vi "Main.vi"   [LabVIEW 2017]
doc: "The start-up VI for our application and the UI"
types:
  T1 = typedef "View Model.ctl" = cluster{"Error Model":T2, "Elevator Model":T3, "Configuration Model":T4, "Shared Model":T5}
  T2 = typedef "Error Model.ctl" = cluster{"Error Event":refnum<user-event>}
  T3 = typedef "Elevator Model.ctl" = cluster{"Elevator Overhead":refnum<data-value>, "Floor Change":refnum<user-event>, "Elevator CMD":refnum<user-event>, "Motion Change":refnum<user-event>, "Direction Change":refnum<user-event>, "Door Position Change":refnum<user-event>, "Emergency Change":refnum<user-event>}
  T4 = typedef "Configuration Model.ctl" = cluster{"Config Change":refnum<user-event>, "Config DVR":refnum<data-value>}
  T5 = typedef "Shared Model.ctl" = cluster{"Stop DVR":refnum<data-value>, "Stop Event":refnum<user-event>}
  T6 = enum32{"invalid app kind", "Development System", "Run Time System", "Student Edition", "Embedded LabVIEW", "Evaluation", "Custom"}
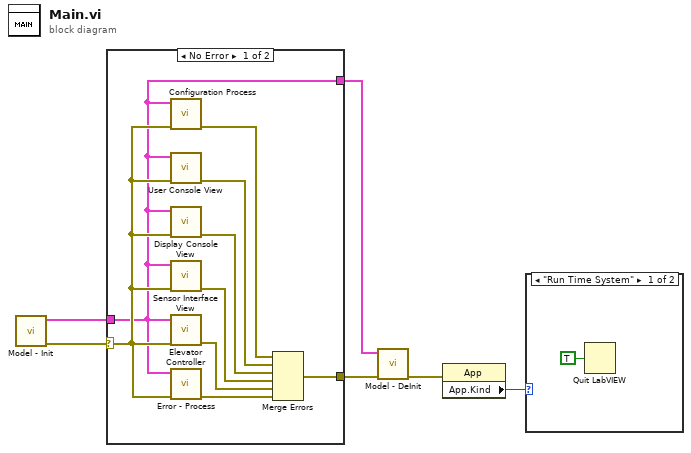
[diagram p0: block diagram]
diagram:
  n1 = call "Model - Init.vi"() -> ("error out"=w6:errorcluster, "View Model"=w5:T1)  [unwired: 10 in]
  n2 = case shown="No Error" w6 {
    selector: w6 -> [w15 w16]
    tunnel: w5 -> [w7 w17]
    tunnel: [w8 w16] -> w4
    tunnel: [w7 w17] -> w3
    frame No Error {
      n3 = call "Configuration Process.vi"("error in (no error)"=w15, "View Model"=w7) -> ("error out"=w9:errorcluster)  [unwired: 9 in]
      n4 = call "User Console View.vi"("error in (no error)"=w15, "View Model"=w7) -> ("error out"=w10:errorcluster)  [unwired: 9 in]
      n5 = call "Display Console View.vi"("error in (no error)"=w15, "View Model"=w7) -> ("error out"=w11:errorcluster)  [unwired: 9 in]
      n6 = call "Sensor Interface View.vi"("error in (no error)"=w15, "View Model"=w7) -> ("error out"=w12:errorcluster)  [unwired: 8 in, 1 out]
      n7 = call "Elevator Controller.vi"("error in (no error)"=w15, "View Model"=w7) -> ("error out"=w13:errorcluster)  [unwired: 9 in]
      n8 = call "Error - Process.vi"("error in (no error)"=w15, "View Model"=w7) -> ("error out"=w14:errorcluster)  [unwired: 9 in]
      n9 = Merge Errors(w9, w10, w11, w12, w13, w14) -> (w8:errorcluster)
    }
    frame Error {
    }
  }
  n10 = call "Model - DeInit.vi"("error in (no error)"=w4, "View Model"=w3) -> ("error out"=w1:errorcluster)  [unwired: 9 in]
  n11 = property class="App"(error in=w1) -> ("App.Kind"=w2:T6)  [unwired: 1 in, 2 out]
  n12 = case shown="\"Run Time System\"" w2 {
    frame "Run Time System" {
      n13 = Quit LabVIEW(quit? (T)=TRUE) -> ()
    }
    frame "Development System", Default {
    }
  }
